vi "Counter with Reset (U64).vi"(2 "Reset?":bool, 7 "Increment":bool) -> (8 "Counter":u64)   [LabVIEW 2014]
panel:
  # "Copyright 2014 Vidrio Technologies\nScanImage 5 software is licensed under the Apache License, Version 2.0 (the \"License\"); you may not use any files contained\nwithin the ScanImage 5 release except in compliance with the License. You may obtain a copy of the License at\n http://www.apache.org/licenses/LICENSE-2.0\nUnless required by applicable law or agreed to in writing, software distributed under the License is distributed on an\n\"AS IS\" BASIS, WITHOUT WARRANTIES OR CONDITIONS OF ANY KIND, either express or implied. See the License for the\n specific language governing permissions and limitations under the License."
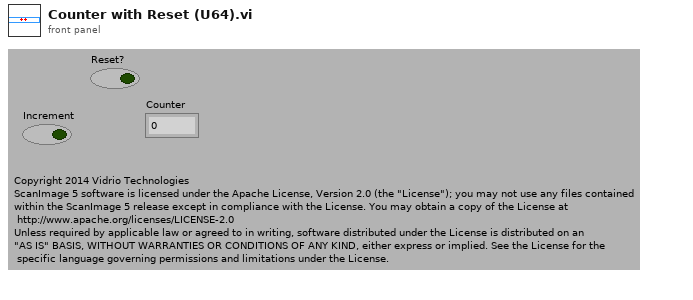
[diagram p1: front panel]
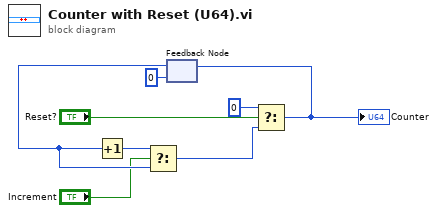
[diagram p0: block diagram]
diagram:
  n1 = feedback #1(u64 0 ("t")) -> (w3:u64)
  n2 = Increment(x=w3) -> (x+1=w4:u64)
  n3 = Select(t=w4, s="Increment", f=w3) -> (s? t:f=w1:u64)
  n4 = Select(t=u64 0, s="Reset?", f=w1) -> (s? t:f=w8:u64)
  "Counter" <- w8
  n5 = feedback-in #1(w8) -> ()
